vi "KE2657A_CommandsGlobal.vi"() -> ()   [LabVIEW 2018, in "KE2657A.lvclass"]
uses:
  KE2657A.lvclass
panel:
  in  "Keithley 2657A GPIB Setup":T1={"Instrument name"="Keithley 2657A", "Command \"Reset\""="smua.reset()", "Command \"Initialise\""="smua.source.func = smua.OUTPUT_DCVOLTS;\n%s;\n%s;\nsmua.source.limiti = %e;\nsmua.measure.adc = smua.ADC_INTEGRATE;\nsmua.measure.nplc = 10;\nsmua.measure.count = 1;\ndisplay.smua.measure.func = display.MEASURE_DCAMPS;\ndisplay.smua.digits = display.DIGITS_6_5;\nsmua.sense = smua.SENSE_LOCAL;", "Command \"Arm\""="smua.source.output = smua.OUTPUT_ON", "Command \"SetVolts\""="smua.source.levelv = %f", "Command \"Compliance?\""="if smua.source.compliance then print(\"1\") else print(\"0\") end", "Command \"Standby\""="smua.source.output = smua.OUTPUT_OFF", "Command \"Read Current\""="print(smua.measure.i())"}
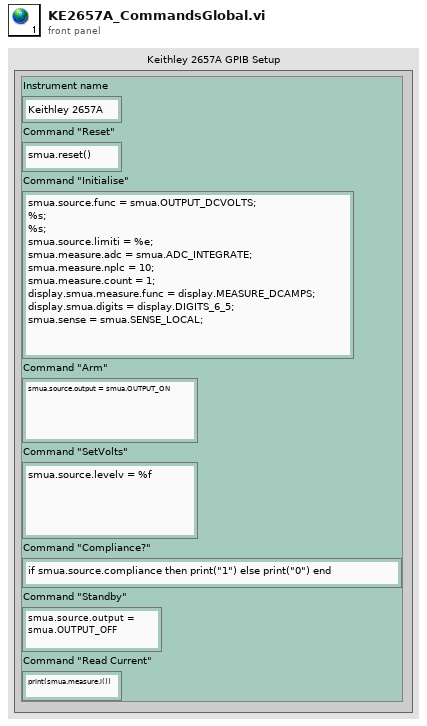
[diagram p1: front panel]
types:
  T1 = cluster{"Instrument name":string, "Command \"Reset\"":string, "Command \"Initialise\"":string, "Command \"Arm\"":string, "Command \"SetVolts\"":string, "Command \"Compliance?\"":string, "Command \"Standby\"":string, "Command \"Read Current\"":string}
diagram:
